vi "Stop Core.vi"(10 "final error code":i32, 11 "Test Actor in":refnum<class "Test Actor.lvclass">) -> (3 "Test Actor out":refnum<class "Test Actor.lvclass">)   [LabVIEW 2020, in "Test.lvlib" / "Test Actor.lvclass"]
doc: "(<B>Filename</B>: Actor Framework.lvlib:Actor.lvclass:Stop Core.vi)\n\nDefines what the actor does before it stops. Use the <B>final error code</B> input to determine whether the actor shut down in response to an error.\n\nBy default, this method does nothing. A descendant class may override it to define behavior, such as shutting down any processes the actor initiated in its override of the Actor Core method."
uses:
  Test Actor.lvclass
  Test Actor.lvclass/Test Actor.ctl
  PPL/HDH.Actor Framework.Core.Sequencer.lvlibp/Sequencer/Sequencer.lvclass
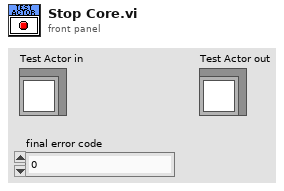
[diagram p1: front panel]
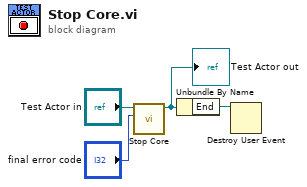
[diagram p0: block diagram]
diagram:
  n1 = call-parent "Stop Core.vi"("final error code"="final error code", "Sequencer in"="Test Actor in") -> ("Sequencer out"=w2:refnum<class "Test Actor.lvclass">)  [unwired: 9 in]
  "Test Actor out" <- w2
  n2 = Unbundle By Name(w2) -> ("End"=w1:refnum<user-event>)
  n3 = Destroy User Event(user event=w1) -> ()  [unwired: 1 in, 1 out]
